vi "Lakeshore218Init.vi"(8 "error in (no error)":errorcluster, 11 "VISA resource name":refnum<visa-resource-name>) -> (0 "error out":errorcluster, 3 "VISA resource name out":refnum<visa-resource-name>)   [LabVIEW 2018]
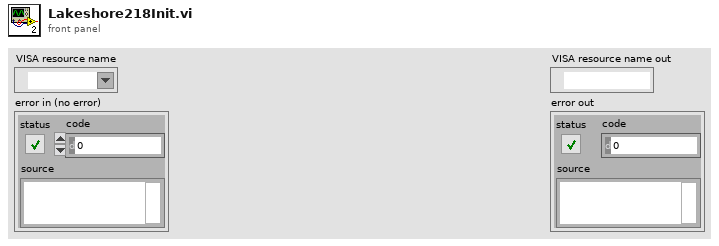
[diagram p1: front panel]
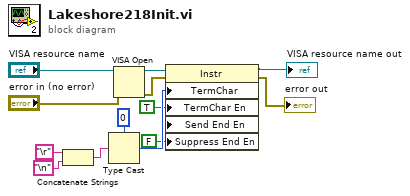
[diagram p0: block diagram]
diagram:
  w4 = TRUE ("Message Based Settings:Termination Character Enable")
  n1 = Concatenate Strings("\r", "\n") -> (w9:string)
  n2 = Type Cast(type=u8 0, x=w9) -> (*(type *) &x=w11:u8)
  n3 = VISA Open(error in (no error)="error in (no error)", VISA resource name="VISA resource name") -> (VISA resource name=w5:refnum<visa-resource-name>, error out=w6:errorcluster)  [unwired: 3 in]
  n4 = property class="Instr"(reference=w5, error in=w6, "TermChar"=w11, "TermChar En"=w4, "Send End En"=w4, "Suppress End En"=FALSE ("Message Based Settings:Suppress End Enable")) -> (reference out=→"VISA resource name out":refnum<visa-resource-name>, error out=→"error out":errorcluster)
